vi "AD_scan.vi"() -> ()   [LabVIEW 2012]
uses:
  Usb_Daq_V52_Dll.dll
panel:
  in  "stop 2":bool
  in  "过采样":i32 min=0 max=7
  out "Numeric":dbl
  out "Waveform Graph":dynamicdata(graph)
  in  "采样频率":i32=1000 min=100 max=100000 step=1
  in  "采样个数":i32=1024 min=512 step=512
  in  "放大倍数":i32 min=0 max=1 step=1
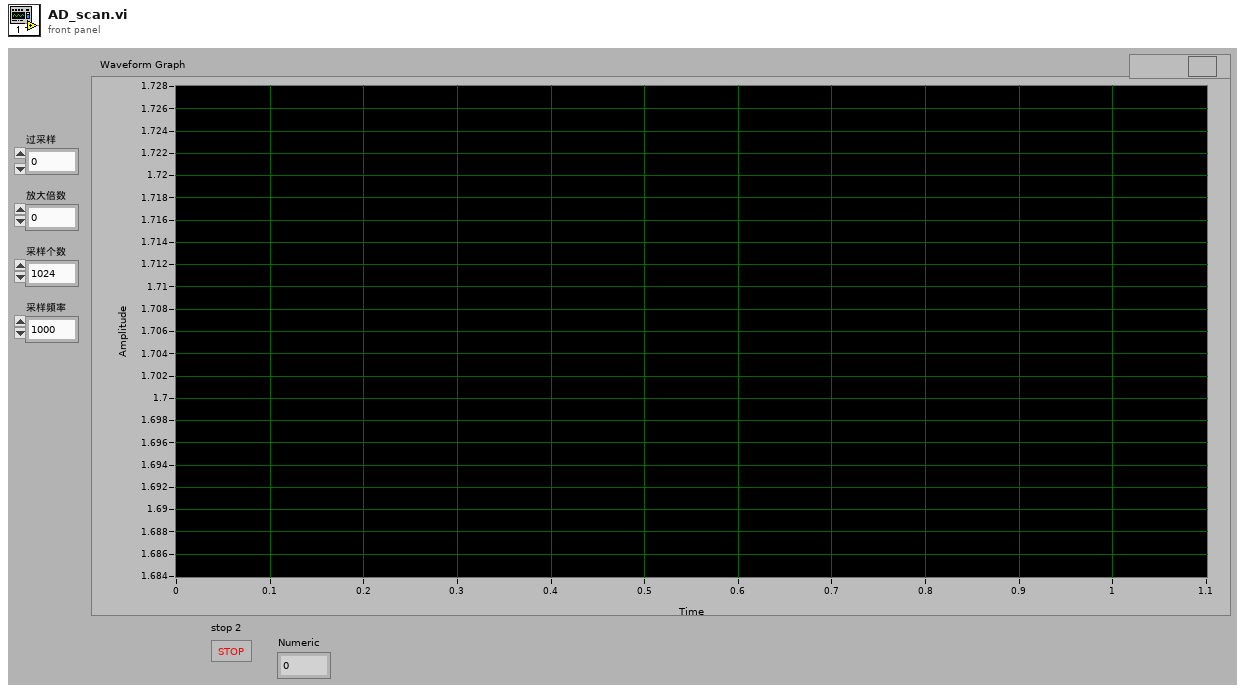
[diagram p1: front panel]
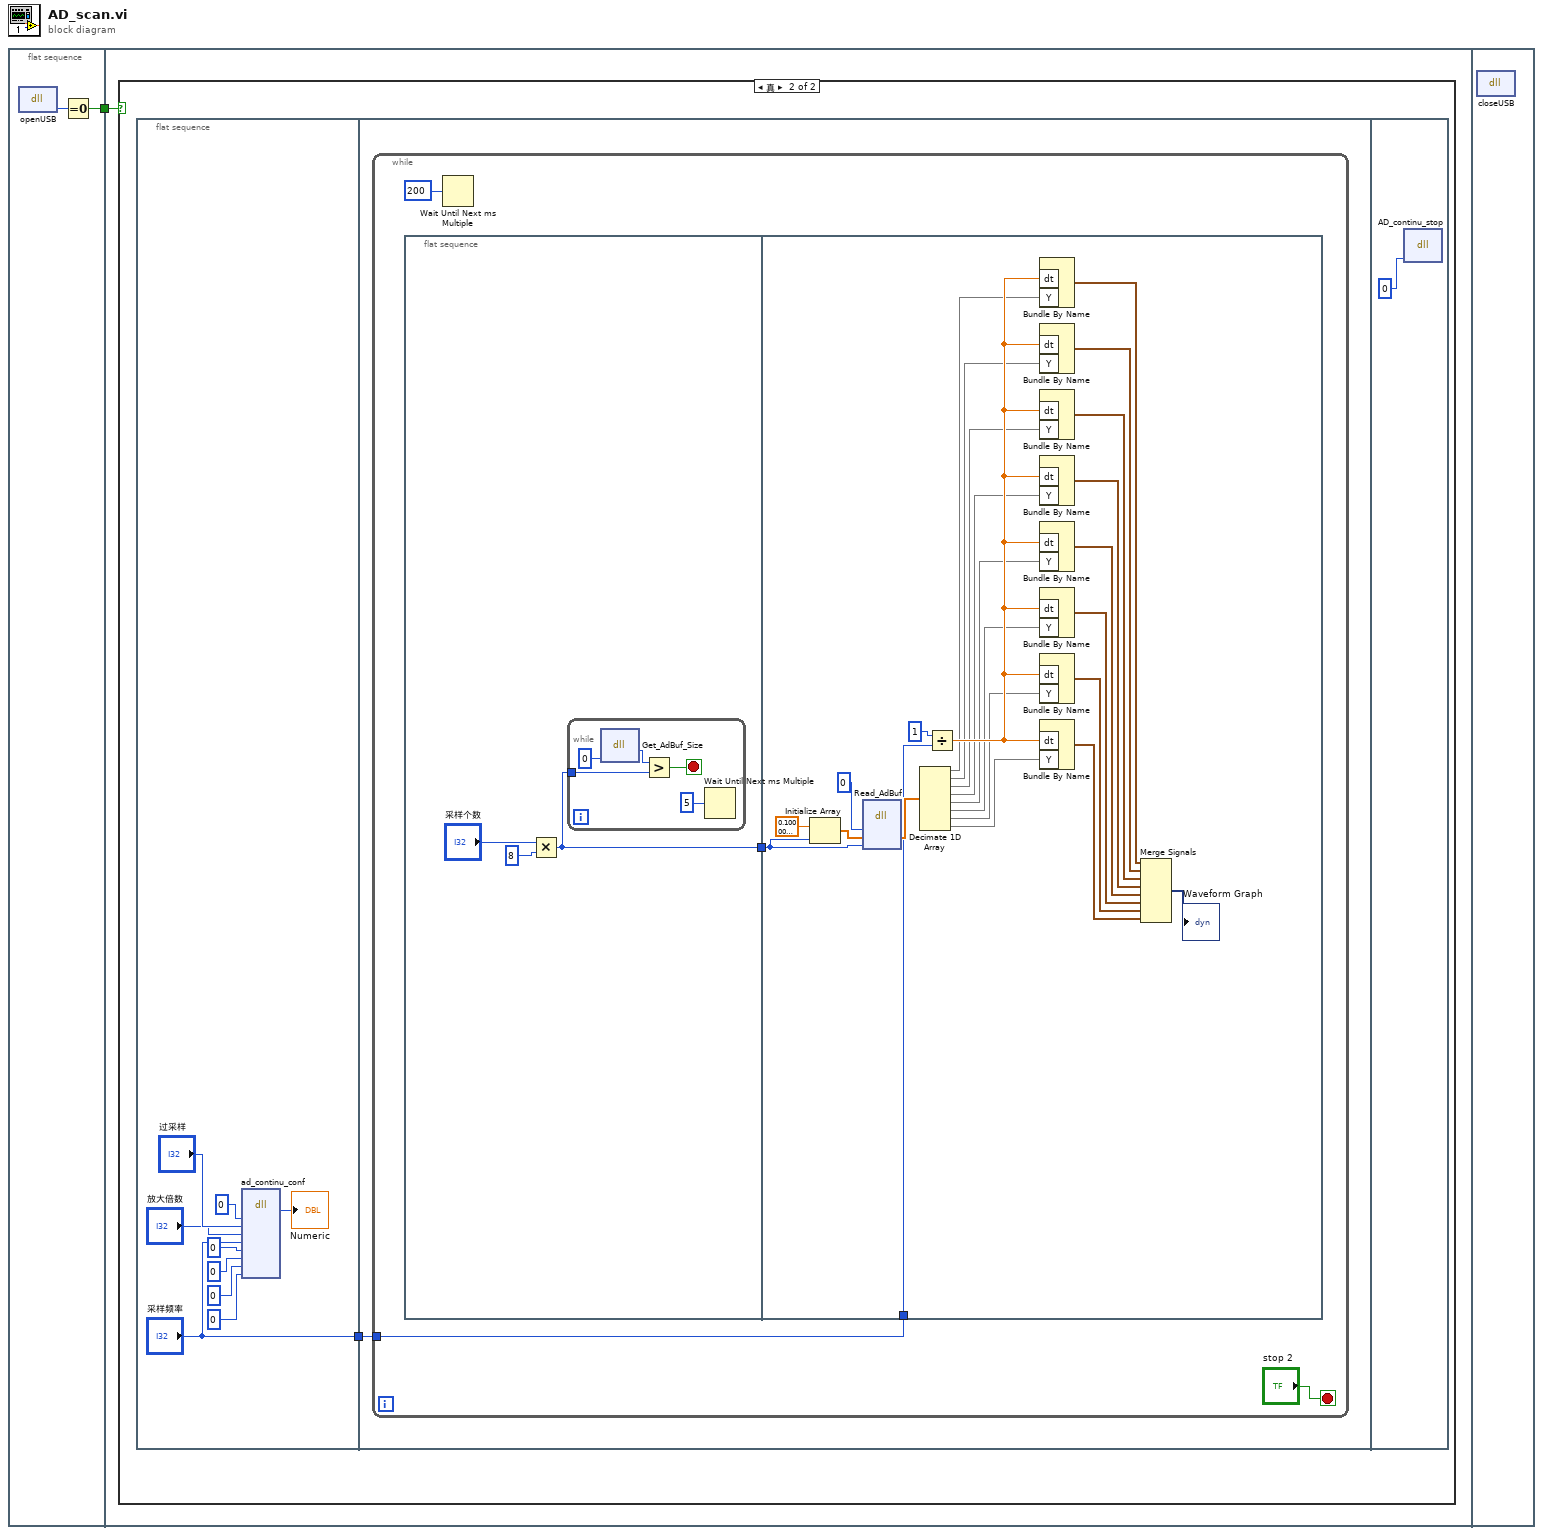
[diagram p0: block diagram]
diagram:
  n1 = flat-sequence {
    tunnel: [w2] -> w1
    tunnel: w1 -> [w4]
    frame #0 {
      n2 = dll-call lib="PTH1labs Ebackup数据采集卡uSB!USB数据采集卡资料HKUSB6203例程labviewUsb_Daq_V52_Dll.dll" fn="openUSB"() -> ("返回类型"=w3:i32)  [unwired: 3 in, 2 out]
      n3 = Equal To 0?(x=w3) -> (x = 0?=w2:bool)
    }
    frame #1 {
      n4 = case shown="真" w4 {
        frame False {
        }
        frame True {
          n5 = flat-sequence {
            tunnel: ["采样频率"] -> w5
            tunnel: w5 -> [w15]
            frame #0 {
              n6 = dll-call lib="PTH1labs Ebackup数据采集卡uSB!USB数据采集卡资料HKUSB6203例程labviewUsb_Daq_V52_Dll.dll" fn="ad_continu_conf"("dev"=0, "ad_os"="过采样", "gain"="放大倍数", "Rate_Sample"="采样频率", "trig_sl"=0, "trig_pol"=0, "clk_sl"=0, "ext_clk_pol"=0) -> ("返回类型"=→"Numeric":i32)  [unwired: 10 in, 3 out]
            }
            frame #1 {
              n7 = while {
                tunnel: w15 -> [w16]
                stop <- "stop 2" stop-if-true
                n8 = flat-sequence {
                  tunnel: [w20] -> w19
                  tunnel: w19 -> [w51]
                  tunnel: w16 -> [w30]
                  frame #0 {
                    n9 = Multiply(x="采样个数", y=8) -> (x*y=w20:i32)
                    n10 = while {
                      tunnel: w20 -> [w25]
                      stop <- w26 stop-if-true
                      n11 = dll-call lib="PTH1labs Ebackup数据采集卡uSB!USB数据采集卡资料HKUSB6203例程labviewUsb_Daq_V52_Dll.dll" fn="Get_AdBuf_Size"("dev"=0) -> ("返回类型"=w27:i32)  [unwired: 3 in, 3 out]
                      n12 = Greater?(x=w27, y=w25) -> (0:w26:bool)
                      n13 = Wait Until Next ms Multiple(millisecond multiple=5) -> ()  [unwired: 1 out]
                    }
                  }
                  frame #1 {
                    n14 = Initialize Array(sgl 0.1, w51) -> (w50:sgl[])
                    n15 = dll-call lib="PTH1labs Ebackup数据采集卡uSB!USB数据采集卡资料HKUSB6203例程labviewUsb_Daq_V52_Dll.dll" fn="Read_AdBuf"("dev"=0, "buf"=w50, "um"=w51) -> ("buf"=w31:sgl[])  [unwired: 3 in, 5 out]
                    n16 = Decimate 1D Array(w31) -> (w32:sgl[], w33:sgl[], w34:sgl[], w35:sgl[], w36:sgl[], w37:sgl[], w38:sgl[], w39:sgl[])
                    n17 = Divide(x=1, y=w30) -> (x/y=w49:dbl)
                    n18 = Bundle By Name ("创建波形")("dt"=w49, "Y"=w32) -> (w41:waveform(sgl))  [unwired: 1 in]
                    n19 = Bundle By Name ("创建波形")("dt"=w49, "Y"=w33) -> (w42:waveform(sgl))  [unwired: 1 in]
                    n20 = Bundle By Name ("创建波形")("dt"=w49, "Y"=w34) -> (w43:waveform(sgl))  [unwired: 1 in]
                    n21 = Bundle By Name ("创建波形")("dt"=w49, "Y"=w35) -> (w44:waveform(sgl))  [unwired: 1 in]
                    n22 = Bundle By Name ("创建波形")("dt"=w49, "Y"=w36) -> (w45:waveform(sgl))  [unwired: 1 in]
                    n23 = Bundle By Name ("创建波形")("dt"=w49, "Y"=w37) -> (w46:waveform(sgl))  [unwired: 1 in]
                    n24 = Bundle By Name ("创建波形")("dt"=w49, "Y"=w38) -> (w47:waveform(sgl))  [unwired: 1 in]
                    n25 = Bundle By Name ("创建波形")("dt"=w49, "Y"=w39) -> (w48:waveform(sgl))  [unwired: 1 in]
                    n26 = Merge Signals(w41, w42, w43, w44, w45, w46, w47, w48) -> (→"Waveform Graph":dynamicdata)
                  }
                }
                n27 = Wait Until Next ms Multiple(millisecond multiple=200) -> ()  [unwired: 1 out]
              }
            }
            frame #2 {
              n28 = dll-call lib="PTH1labs Ebackup数据采集卡uSB!USB数据采集卡资料HKUSB6203例程labviewUsb_Daq_V52_Dll.dll" fn="AD_continu_stop"("dev"=0) -> ()  [unwired: 3 in, 4 out]
            }
          }
        }
      }
    }
    frame #2 {
      n29 = dll-call lib="PTH1labs Ebackup数据采集卡uSB!USB数据采集卡资料HKUSB6203例程labviewUsb_Daq_V52_Dll.dll" fn="closeUSB"() -> ()  [unwired: 3 in, 3 out]
    }
  }
